vi "Teleop.vi"(10 "Match Info":T1={"Autonomous Elapsed Seconds"=0.0, "TeleOp Elapsed Seconds"=0.0, "Disabled Elapsed Seconds"=0.0, "Visited Autonomous"=FALSE, "Visited TeleOp"=FALSE, "Visited Disabled"=FALSE, "Autonomous Settings"={"Autonomous Style"=enum."Independent", "VI Refnum"=refnum}}, 11 "Call Context":T2) -> ()   [LabVIEW 2016]
doc: "This VI is called for each TeleOp packet received from the DS where the robot is not disabled. It is often used to read from the joysticks and update I/O or to update setpoints for timed control loops. It should complete and return within 20 milliseconds or it may miss DS packets."
uses:
  <vilib>/Rock Robotics/WPI/DriverStation/WPI_DriverStationDerivedRobotMode.ctl
  <vilib>/Rock Robotics/WPI/DriverStation/WPI_DriverStationMatch Info.ctl
  <vilib>/Rock Robotics/WPI/Solenoid/WPI_SolenoidValue.ctl
  <vilib>/Rock Robotics/WPI/Utilities/WPI_GetSetVariantRefNum.vi
  <vilib>/Rock Robotics/WPI/Solenoid/WPI_SolenoidSetEnum.vi
  Robot Global Data.vi
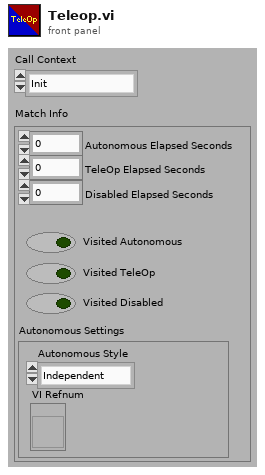
[diagram p1: front panel]
types:
  T1 = typedef "WPI_DriverStationMatch Info.ctl" = cluster{"Autonomous Elapsed Seconds":dbl, "TeleOp Elapsed Seconds":dbl, "Disabled Elapsed Seconds":dbl, "Visited Autonomous":bool, "Visited TeleOp":bool, "Visited Disabled":bool, "Autonomous Settings":cluster{"Autonomous Style":enum16{"Iterative", "Independent"}, "VI Refnum":refnum<vi>}}
  T2 = typedef "WPI_DriverStationDerivedRobotMode.ctl" = enum16{"Init", "Execute", "Stop"}
  T3 = typedef "WPI_SolenoidValue.ctl" = enum16{"Off", "On", "Forward", "Reverse"}
  T4 = typedef "WPI_JoystickDevRef.ctl" = cluster{"Device":T5}
  T5 = typedef "WPI_JoystickDeviceEnum.ctl" = enum16{"USB 0", "USB 1", "USB 2", "USB 3", "USB 4", "USB 5"}
  T6 = typedef "WPI_SolenoidDevRef.ctl" = cluster{"DevStatus":errorcluster, "Pneumatics Control Module":u8, "Forward Solenoid Channel":T7, "Reverse Solenoid Channel":T7}
  T7 = typedef "WPI_SolenoidChannel.ctl" = enum8{"Solenoid 0", "Solenoid 1", "Solenoid 2", "Solenoid 3", "Solenoid 4", "Solenoid 5", "Solenoid 6", "Solenoid 7", "Invalid"}
  T8 = typedef "WPI_RobotDriveDevRef.ctl" = cluster{"DevStatus":errorcluster, "Motors[]":T9[], "Square Inputs":bool, "Max Output":dbl}
  T9 = typedef "WPI_MotorControlDeviceRef.ctl" = cluster{"DeviceStatus":errorcluster, "Type":T10, "PWM":cluster{"PWM Channel":T11, "DeadBand":T12}, "CAN":cluster{"Device Number":u8, "SetOutput VI Ref":variant, "GetOutput VI Ref":variant, "Enable VI Ref":variant, "Disable VI Ref":variant, "Data":variant}, "Invert":bool}
  T10 = typedef "WPI_MotorControlType.ctl" = enum16{"PWM", "CAN"}
  T11 = typedef "FPGA_DIOPWMChannel.ctl" = enum8{"PWM 0", "PWM 1", "PWM 2", "PWM 3", "PWM 4", "PWM 5", "PWM 6", "PWM 7", "PWM 8", "PWM 9", "PWM MXP 0", "PWM MXP 1", "PWM MXP 2", "PWM MXP 3", "PWM MXP 4", "PWM MXP 5", "PWM MXP 6", "PWM MXP 7", "PWM MXP 8", "PWM MXP 9", "Invalid"}
  T12 = typedef "WPI_PWMDeadband.ctl" = cluster{"Name":string, "maxPositivePwm":i32, "minPositivePwm":i32, "centerPwm":i32, "maxNegativePwm":i32, "minNegativePwm":i32, "angularRange":u16}
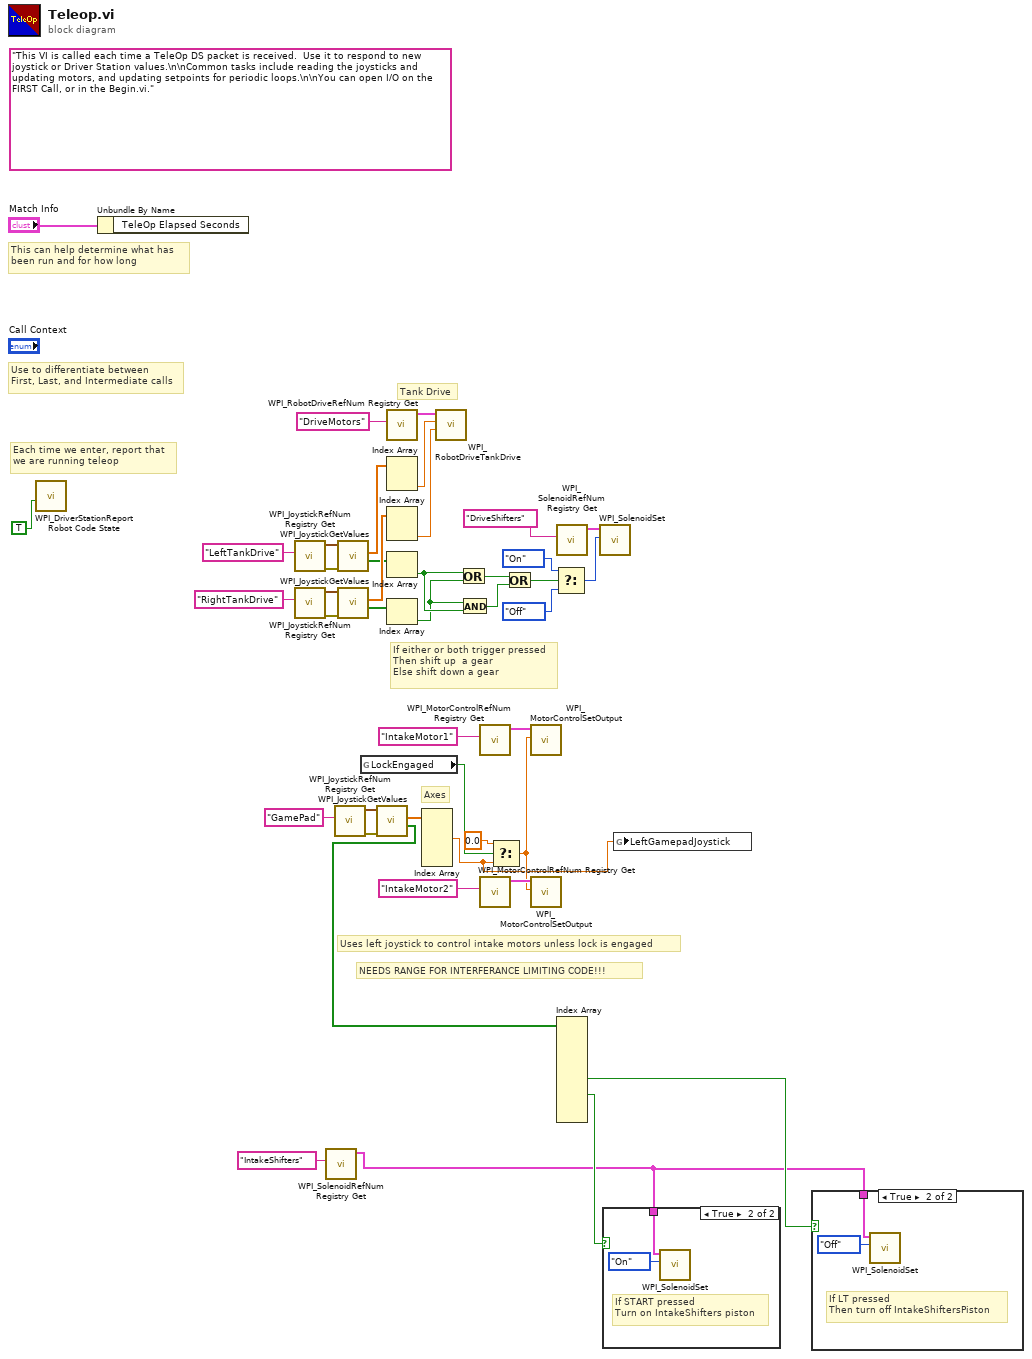
[diagram p0: block diagram]
diagram:
  (unwired) "This VI is called each time a TeleOp DS packet is received.  Use it to respond to new joystick or Driver Station values.\n\nCommon tasks include reading the joysticks and updating motors, and updating setpoints for periodic loops.\n\nYou can open I/O on the FIRST Call, or in the Begin.vi."
  # "NEEDS RANGE FOR INTERFERANCE LIMITING CODE!!!"
  # "Uses left joystick to control intake motors unless lock is engaged"
  # "Axes"
  # "Tank Drive"
  # "If either or both trigger pressed\nThen shift up  a gear\nElse shift down a gear"
  # "Each time we enter, report that\nwe are running teleop"
  # "Use to differentiate between\nFirst, Last, and Intermediate calls"
  # "This can help determine what has\nbeen run and for how long"
  n1 = call <vilib>:"WPI_DriverStationReport Robot Code State.vi"("TeleOp"=TRUE ("Autonomous")) -> ()  [unwired: 10 in, 1 out]
  n2 = Unbundle By Name("Match Info") -> ()  [unwired: 1 out]
  n3 = call <vilib>:"WPI_JoystickRefNum Registry Get.vi"("refnum name"="LeftTankDrive") -> ("error out"=w41:errorcluster, "JoystickDevRef"=w40:T4)  [unwired: 9 in]
  n4 = call <vilib>:"WPI_JoystickRefNum Registry Get.vi"("refnum name"="RightTankDrive") -> ("error out"=w37:errorcluster, "JoystickDevRef"=w36:T4)  [unwired: 9 in]
  n5 = call <vilib>:"WPI_SolenoidRefNum Registry Get.vi"("refnum name"="IntakeShifters") -> ("SolenoidDevRef"=w2:T6)  [unwired: 9 in, 1 out]
  n6 = call <vilib>:"WPI_JoystickRefNum Registry Get.vi"("refnum name"="GamePad") -> ("error out"=w17:errorcluster, "JoystickDevRef"=w16:T4)  [unwired: 9 in]
  n7 = call <vilib>:"WPI_JoystickGetValues.vi"("error in (no error)"=w41, "JoystickDevRef"=w40) -> ("Buttons"=w28:bool[], "Axes"=w38:dbl[])  [unwired: 5 in, 3 out]
  n8 = call <vilib>:"WPI_JoystickGetValues.vi"("error in (no error)"=w37, "JoystickDevRef"=w36) -> ("Buttons"=w29:bool[], "Axes"=w35:dbl[])  [unwired: 5 in, 3 out]
  n9 = global read "Robot Global Data.vi" "LockEngaged"() -> (w11:bool)
  n10 = call <vilib>:"WPI_JoystickGetValues.vi"("error in (no error)"=w17, "JoystickDevRef"=w16) -> ("Buttons"=w4:bool[], "Axes"=w14:dbl[])  [unwired: 5 in, 3 out]
  n11 = call <vilib>:"WPI_RobotDriveRefNum Registry Get.vi"("refnum name"="DriveMotors") -> ("RobotDriveDevRef"=w39:T8)  [unwired: 9 in, 1 out]
  n12 = Index Array(array=w38) -> (element #2=w33:dbl)  [unwired: 2 in, 1 out]
  n13 = Index Array(array=w35) -> (element #2=w34:dbl)  [unwired: 2 in, 1 out]
  n14 = Index Array(array=w28) -> (element=w27:bool)  [unwired: 1 in]
  n15 = Index Array(array=w29) -> (element=w26:bool)  [unwired: 1 in]
  n16 = Index Array(array=w14) -> (element #2=w1:dbl)  [unwired: 5 in, 4 out]
  n17 = call <vilib>:"WPI_RobotDriveTankDrive.vi"("Right axis value"=w34, "Left axis value"=w33, "RobotDriveDevRef"=w39) -> ()  [unwired: 6 in, 3 out]
  n18 = Or(x=w27, y=w26) -> (x .or. y?=w25:bool)
  n19 = And(x=w26, y=w27) -> (x .and. y?=w24:bool)
  n20 = call <vilib>:"WPI_MotorControlRefNum Registry Get.vi"("refnum name"="IntakeMotor1") -> ("MotorControlDevRef"=w9:T9)  [unwired: 9 in, 1 out]
  n21 = call <vilib>:"WPI_MotorControlRefNum Registry Get.vi"("refnum name"="IntakeMotor2") -> ("MotorControlDevRef"=w8:T9)  [unwired: 9 in, 1 out]
  n22 = Select(t=0.0, s=w11, f=w1) -> (s? t:f=w7:dbl)
  n23 = Or(x=w25, y=w24) -> (x .or. y?=w22:bool)
  n24 = call <vilib>:"WPI_MotorControlSetOutput.vi"("Output"=w7, "MotorControlDevRef"=w9) -> ()  [unwired: 7 in, 3 out]
  n25 = call <vilib>:"WPI_MotorControlSetOutput.vi"("Output"=w7, "MotorControlDevRef"=w8) -> ()  [unwired: 7 in, 3 out]
  n26 = Select(t=WPI_SolenoidValue."On" ("Value"), s=w22, f=WPI_SolenoidValue."Off" ("Value")) -> (s? t:f=w19:T3)
  n27 = call <vilib>:"WPI_SolenoidRefNum Registry Get.vi"("refnum name"="DriveShifters") -> ("SolenoidDevRef"=w23:T6)  [unwired: 9 in, 1 out]
  n28 = Index Array(array=w4) -> (element #6=w6:bool, element #8=w5:bool)  [unwired: 11 in, 9 out]
  n29 = call-poly <vilib>:"WPI_SolenoidSet.vi"("Value"=w19, "SolenoidDevRef"=w23) -> ()  [unwired: 8 in, 2 out]
  n30 = case shown="True" w5 {
    tunnel: w2 -> [_ w44]
    frame False {
    }
    frame True {
      # "If START pressed\nTurn on IntakeShifters piston"
      n31 = call-poly <vilib>:"WPI_SolenoidSet.vi"("Value"=WPI_SolenoidValue."On", "SolenoidDevRef"=w44) -> ()  [unwired: 8 in, 2 out]
    }
  }
  n32 = global write "Robot Global Data.vi" "LeftGamepadJoystick"(w1) -> ()
  n33 = case shown="True" w6 {
    tunnel: w2 -> [_ w46]
    frame False {
    }
    frame True {
      # "If LT pressed\nThen turn off IntakeShiftersPiston"
      n34 = call-poly <vilib>:"WPI_SolenoidSet.vi"("Value"=WPI_SolenoidValue."Off", "SolenoidDevRef"=w46) -> ()  [unwired: 8 in, 2 out]
    }
  }
